vi "ScheduleUnlimitedTimeSlotsforRobot.vi"(6 "excelList":string[][](array[string])=[["21:31", "681_2602_1", "1", "2,5", "3"], ["21:32", "681_2620_Intro_note", "1", "2,5", "3"], ["21:33", "681CIMG1259_2620_2nd_Contact_calls", "1", "2,5", "3"], ["21:34", "681CIMG1259_2620_2nd_headMOV1_normTo7", "1", "2,5", "3"]], 7 "Timer active":bool=TRUE, 9 "current time":timestamp=timestamp(3646064105.849446 s since 1904-01-01)) -> (0 "activation":bool, 1 "Array 2":string[](array[string]), 3 "current time":timestamp=timestamp(3646064100 s since 1904-01-01), 4 "output 1":timestamp=timestamp(3646064040 s since 1904-01-01))   [LabVIEW 2014]
panel:
  out "Array":bool[](array[boolean])
  out "concatenated string":string="21:3415/07/2019"
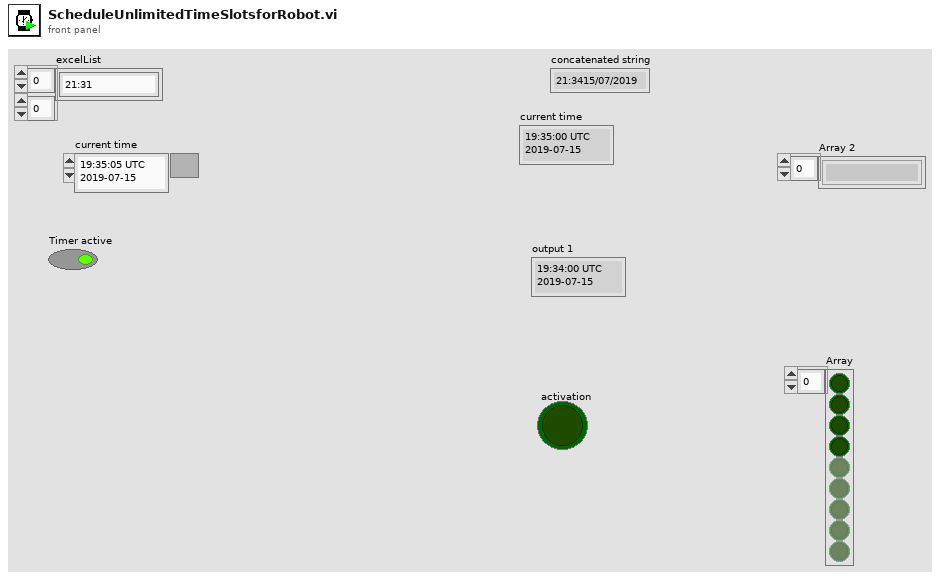
[diagram p1: front panel]
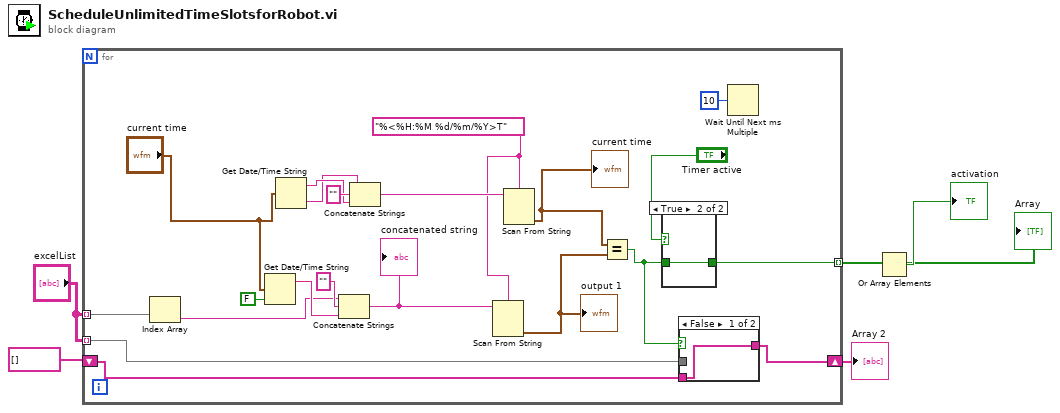
[diagram p0: block diagram]
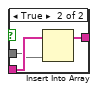
[diagram p2: hidden frame]
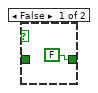
[diagram p3: hidden frame]
diagram:
  n1 = for {
    tunnel: [w11] -> w4 mode=indexing
    tunnel: "excelList" -> [w10] mode=indexing
    shift-right: [w6] -> w1
    shift-left: string[] [] -> [w7]
    tunnel: "excelList" -> [w8] mode=indexing
    w18 = "%<%H:%M %d/%m/%Y>T" ("format string")
    n2 = Index Array(array=w10) -> (element=w12:string)  [unwired: 1 in]
    n3 = Get Date/Time String(seconds (now)="current time", want seconds? (F)=FALSE) -> (date string=w16:string)  [unwired: 1 in, 1 out]
    n4 = Get Date/Time String(seconds (now)="current time") -> (date string=w21:string, time string=w20:string)  [unwired: 2 in]
    n5 = Concatenate Strings(w12, "" ("string"), w16) -> (w25:string)
    "concatenated string" <- w25
    n6 = Concatenate Strings(w20, "" ("string"), w21) -> (w22:string)
    n7 = Scan From String(format string=w18, input string=w25) -> (output 1=w24:timestamp)  [unwired: 3 in, 3 out]
    "output 1" <- w24
    n8 = Scan From String(format string=w18, input string=w22) -> (output 1=w17:timestamp)  [unwired: 3 in, 3 out]
    "current time" <- w17
    n9 = Equal?(x=w17, y=w24) -> (x = y?=w9:bool)
    n10 = case shown="True" "Timer active" {
      tunnel: w9 -> [_ w32]
      tunnel: [FALSE w32] -> w11
      frame False {
      }
      frame True {
      }
    }
    n11 = case shown="False" w9 {
      tunnel: w8 -> [_ w29]
      tunnel: w7 -> [w27 w30]
      tunnel: [w27 w28] -> w6
      frame False {
      }
      frame True {
        n12 = Insert Into Array(array=w30, new element=w29) -> (w28:string[])  [unwired: 1 in]
      }
    }
    n13 = Wait Until Next ms Multiple(millisecond multiple=u32 10) -> ()  [unwired: 1 out]
  }
  "Array" <- w4
  "Array 2" <- w1
  n14 = Or Array Elements(Boolean array=w4) -> (logical OR=→"activation":bool)
